vi "countdown.vi"(1 "buffer in":string) -> (0 "countdown":dbl)   [LabVIEW 2016]
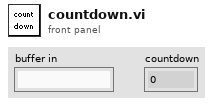
[diagram p1: front panel]
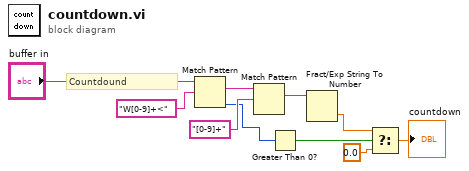
[diagram p0: block diagram]
diagram:
  # "Countdound"
  n1 = Match Pattern(string="buffer in", regular expression="W[0-9]+<") -> (match substring=w5:string, offset past match=w1:i32)  [unwired: 1 in, 2 out]
  n2 = Match Pattern(string=w5, regular expression="[0-9]+") -> (match substring=w6:string)  [unwired: 1 in, 3 out]
  n3 = Greater Than 0?(x=w1) -> (x > 0?=w2:bool)
  n4 = Fract/Exp String To Number(string=w6) -> (number=w7:dbl)  [unwired: 3 in, 1 out]
  n5 = Select(t=w7, s=w2, f=0.0) -> (s? t:f=→"countdown":dbl)
